vi "Dequeue Message.vi"(8 "error in (no error)":errorcluster) -> (0 "error out":errorcluster, 2 "output cluster":T1, 3 "queue out":refnum<queue>)   [LabVIEW 2014, in "User Module.lvlib"]
uses:
  User Module.lvlib
  Message.ctl
  Queue FGV.ctl
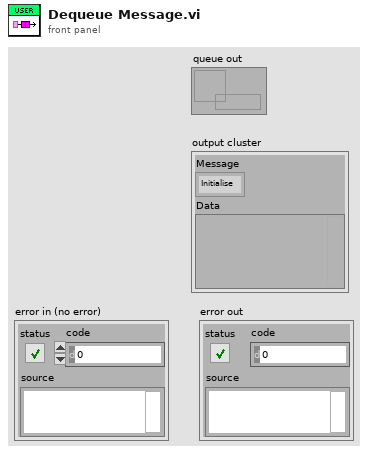
[diagram p1: front panel]
types:
  T1 = typedef "User Module.lvlib/Message.ctl" = cluster{"Message":enum16{"Initialise", "Error", "Close"}, "Data":variant}
  T2 = typedef "User Module.lvlib/Queue FGV.ctl" = enum16{"Set", "Get", "Release"}
  T3 = typedef "User Module.lvlib/User Message.ctl" = cluster{"Message":enum16{"Initialise", "Error", "Close"}, "Data":variant}
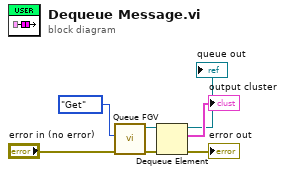
[diagram p0: block diagram]
diagram:
  n1 = call "Queue FGV.vi"("error in (no error)"="error in (no error)", "Action"=Queue_FGV."Get") -> ("error out"=w5:errorcluster, "Queue Out"=w6:refnum<queue>)  [unwired: 8 in]
  n2 = Dequeue Element(queue=w6, error in (no error)=w5) -> (queue out=→"queue out":refnum<queue>, element=→"output cluster":T3, error out=→"error out":errorcluster)  [unwired: 1 in, 1 out]
